vi "SetScale.vi"(10 "Scale":refnum<class "Scale_PiecedLinear.lvclass">, 11 "Sig_AI in":refnum<class "AI.lvclass">) -> (3 "Sig_AI out":refnum<class "AI.lvclass">)   [LabVIEW 2019, in "AI.lvclass"]
uses:
  AI.lvclass
  PiecedLinearScale_class/Scale_PiecedLinear.lvclass
  AI.lvclass/AI.ctl
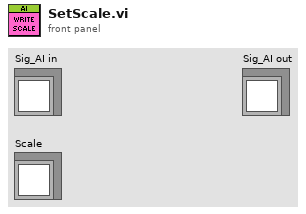
[diagram p1: front panel]
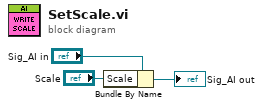
[diagram p0: block diagram]
diagram:
  n1 = Bundle By Name(cluster="Sig_AI in", "Scale"="Scale") -> (→"Sig_AI out":refnum<class "AI.lvclass">)
